vi "EndRotation.vi"(6 "Rotation(Deg)":sgl, 8 "error in (no error)":errorcluster, 9 "dyTranslation":sgl, 10 "dxTranslation":sgl, 11 ".NET Refnum in":refnum<k24>) -> (0 "error out":errorcluster, 3 ".NET Refnum out":refnum<k24>)   [LabVIEW 2020, in "LcPictureBox.lvclass"]
uses:
  LcPictureBox.lvclass
  System.Drawing
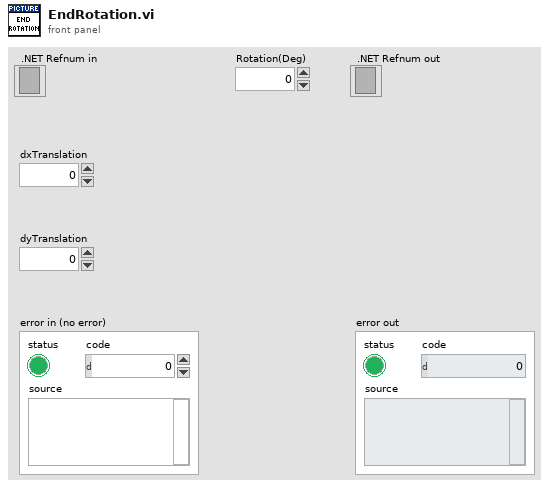
[diagram p1: front panel]
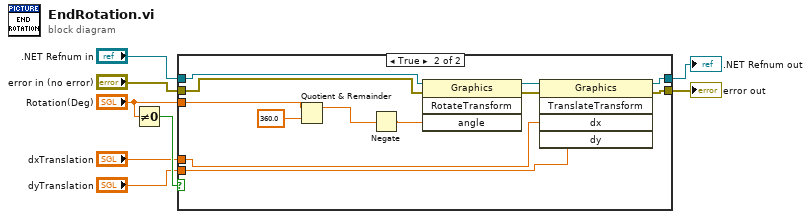
[diagram p0: block diagram]
diagram:
  n1 = Not Equal To 0?(x="Rotation(Deg)") -> (x != 0?=w8:bool)
  n2 = case shown="True" w8 {
    tunnel: ".NET Refnum in" -> [w9 w22]
    tunnel: "error in (no error)" -> [w10 w21]
    tunnel: "Rotation(Deg)" -> [_ w12]
    tunnel: [w10 w16] -> w5
    tunnel: "dxTranslation" -> [_ w18]
    tunnel: "dyTranslation" -> [_ w17]
    tunnel: [w9 w15] -> w6
    frame False {
    }
    frame True {
      n3 = Quotient & Remainder(x=w12, y=360.0) -> (x-y*floor(x/y)=w11:dbl)  [unwired: 1 out]
      n4 = Negate(x=w11) -> (-x=w14:dbl)
      n5 = invoke class="Graphics" method="RotateTransform"(reference=w22, error in=w21, "angle"=w14) -> (reference out=w20:refnum<k24>, error out=w19:errorcluster)  [unwired: 1 in, 2 out]
      n6 = invoke class="Graphics" method="TranslateTransform"(reference=w20, error in=w19, "dx"=w18, "dy"=w17) -> (reference out=w15:refnum<k24>, error out=w16:errorcluster)  [unwired: 1 in, 3 out]
    }
  }
  ".NET Refnum out" <- w6
  "error out" <- w5
